vi "I2C_Send_1_Byte_DAQ.vi"(2 "Byte_To_Send":u8 format="%02x") -> ()   [LabVIEW 2022 SP3]
doc: "Petrus Prins 7 June 2026"
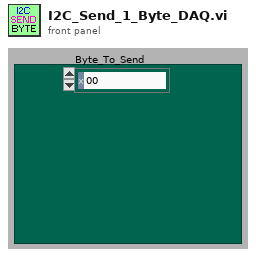
[diagram p1: front panel]
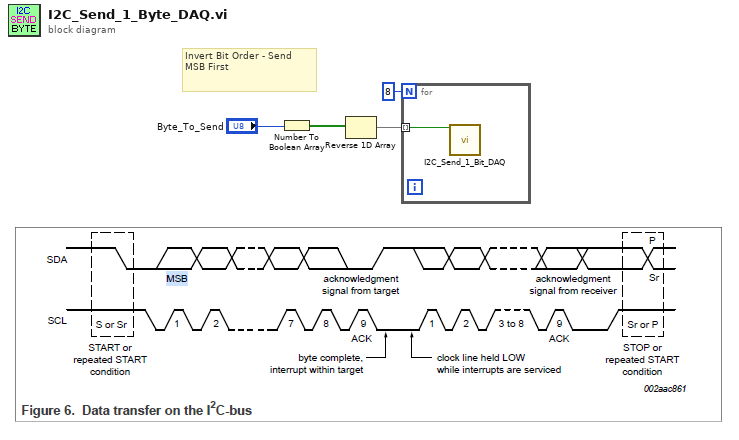
[diagram p0: block diagram]
diagram:
  # "Invert Bit Order - Send MSB First"
  n1 = Number To Boolean Array(number="Byte_To_Send") -> (Boolean array=w3:bool[])
  n2 = Reverse 1D Array(array=w3) -> (reversed array=w1:bool[])
  n3 = for {
    N: 8 -> [_]
    tunnel: w1 -> [w5] mode=indexing
    n4 = call "I2C_Send_1_Bit_DAQ.vi"("Data_Bit"=w5) -> ()  [unwired: 2 in]
  }
